vi "parallel loops.vi"() -> ()   [LabVIEW 2020]
panel:
  in  "Stop":bool
  out "Waveform Chart 2":dbl(graph)
  out "Waveform Chart":dbl(graph)
  out "sin(x) 2":dbl
  out "sin(x)":dbl
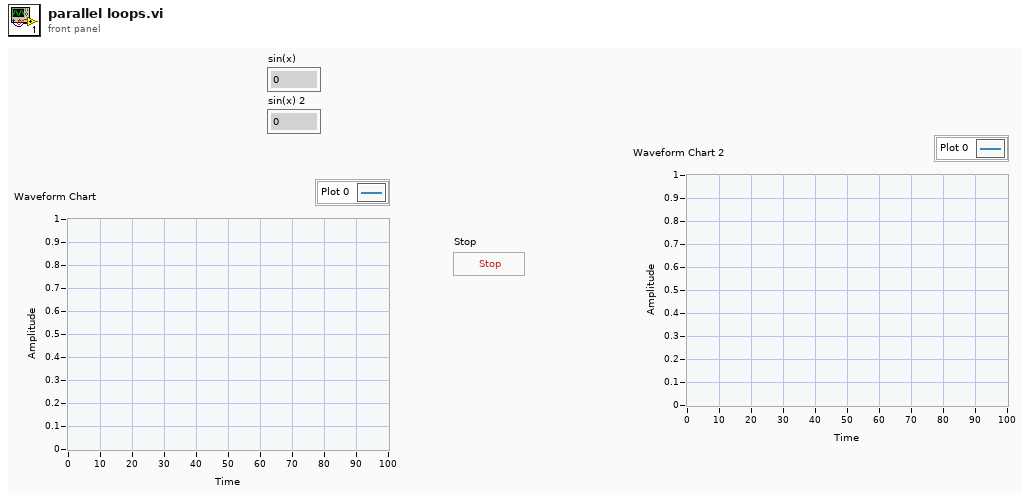
[diagram p1: front panel]
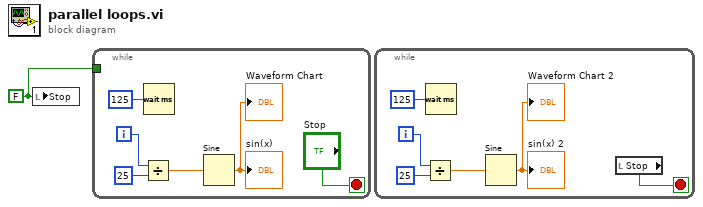
[diagram p0: block diagram]
diagram:
  w1 = FALSE ("Stop")
  n1 = local write "Stop"(w1) -> ()
  n2 = while {
    tunnel: w1 -> [_]
    i -> [w5]
    stop <- "Stop" stop-if-true
    n3 = Divide(x=w5, y=25) -> (x/y=w7:dbl)
    n4 = Wait (ms)(milliseconds to wait=u32 125) -> ()  [unwired: 1 out]
    n5 = Sine(x=w7) -> (sin(x)=→"sin(x)" →"Waveform Chart":dbl)
  }
  n6 = while {
    i -> [w11]
    stop <- w8 stop-if-true
    n7 = Divide(x=w11, y=25) -> (x/y=w13:dbl)
    n8 = Wait (ms)(milliseconds to wait=u32 125) -> ()  [unwired: 1 out]
    n9 = Sine(x=w13) -> (sin(x)=→"sin(x) 2" →"Waveform Chart 2":dbl)
    n10 = local read "Stop"() -> (w8:bool)
  }
